vi "Build Wiring Spec.vi"(8 "error in (no error)":errorcluster, 10 "References":T1) -> (0 "error out":errorcluster, 4 "Wiring Spec":T2)   [LabVIEW 2023, in "Message Maker.lvclass"]
doc: "Figures out the wiring spec for the new message. This wiring spec is used to build the new message\n\nAuthor: Derek Trepanier\nCopyright: MGI 2015"
uses:
  Message Maker.lvclass
  Message Maker.lvclass/Message Maker.ctl
  <vilib>/Utility/VariantDataType/VariantType.lvlib
  Wiring Spec.ctl
  Connector Pane Position.ctl
  Scripting Refs.ctl
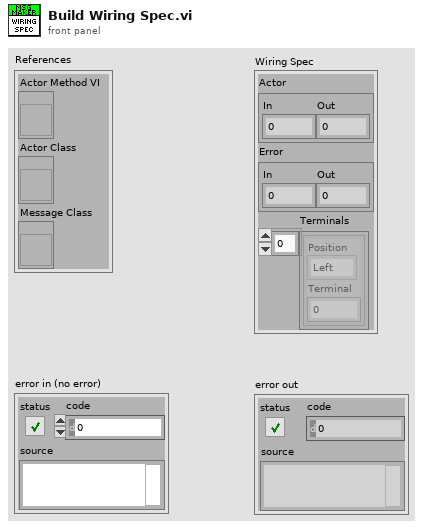
[diagram p1: front panel]
types:
  T1 = typedef "Message Maker.lvclass/Scripting Refs.ctl" = cluster{"Actor Method VI":refnum<vi>, "Actor Class":refnum<vi>, "Message Class":refnum<vi>}
  T2 = typedef "Message Maker.lvclass/Wiring Spec.ctl" = cluster{"Actor":cluster{"In":i32, "Out":i32}, "Error":cluster{"In":i32, "Out":i32}, "Terminals":cluster{"Position":T3, "Terminal":i32}[]}
  T3 = typedef "Message Maker.lvclass/Connector Pane Position.ctl" = enum16{"Left", "Top", "Bottom", "Right"}
  T4 = cluster{"Actor":cluster{"In":i32, "Out":i32}, "Error":cluster{"In":i32, "Out":i32}, "Left":cluster{"Position":i16, "Terminal":i32}[], "Bottom":cluster{"Position":i16, "Terminal":i32}[], "Right":cluster{"Position":i16, "Terminal":i32}[], "Top":cluster{"Position":i16, "Terminal":i32}[]}
  T5 = enum16{"Invalid Wire Rule", "Required", "Recommended", "Optional", "Dynamic Dispatch"}[]
  T6 = typedef "LVRectTypeDef.ctl" = cluster{"Left":i16, "Top":i16, "Right":i16, "Bottom":i16}
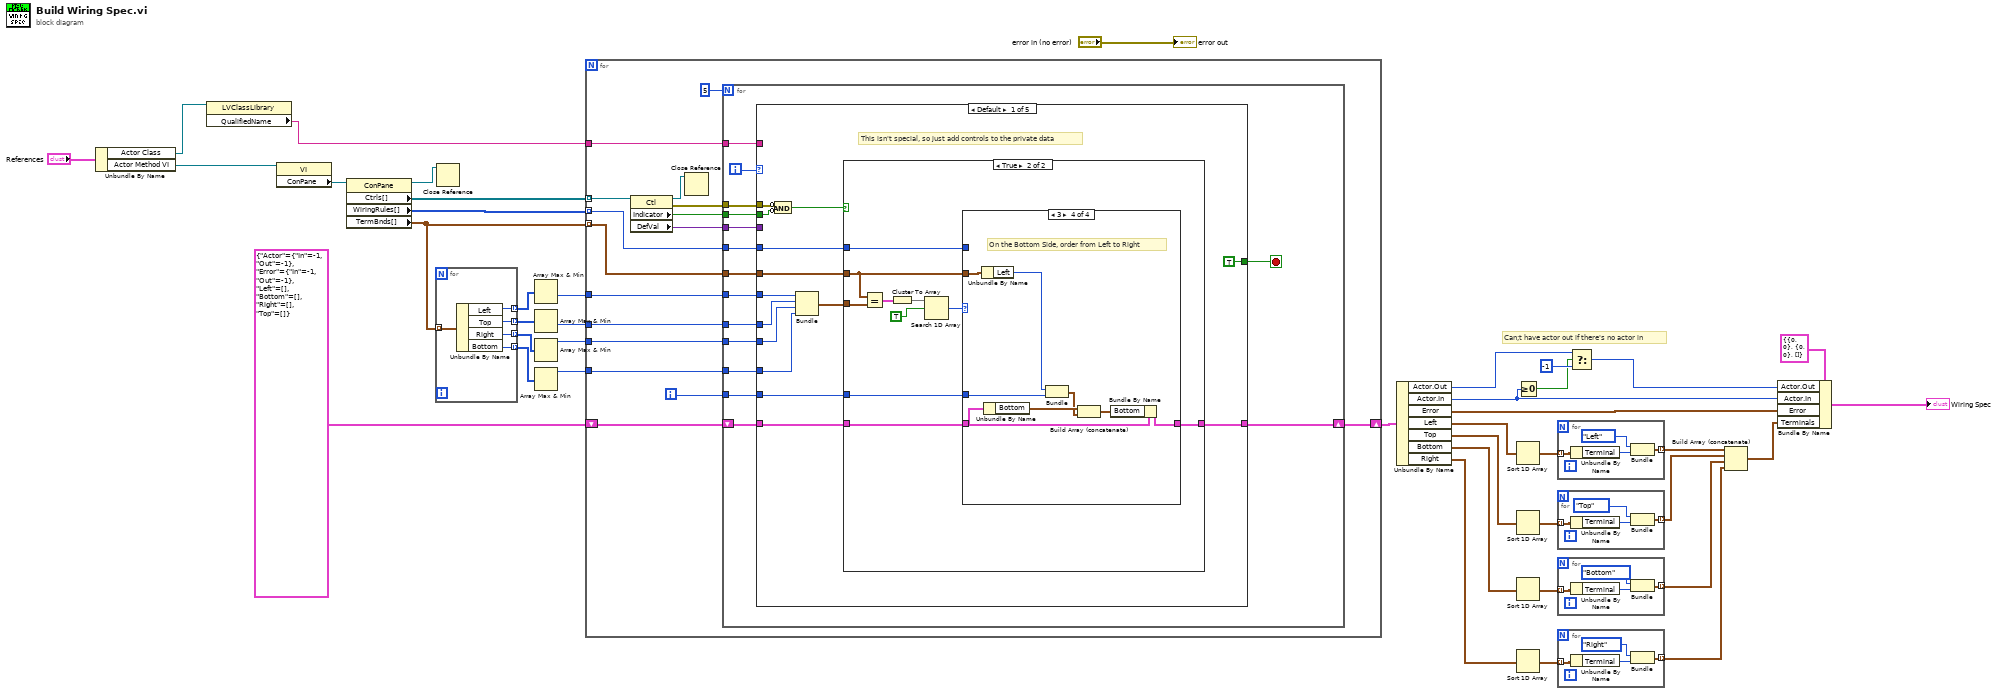
[diagram p0: block diagram]
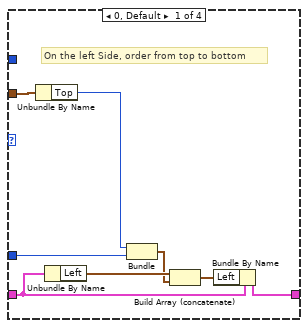
[diagram p3: hidden frame]
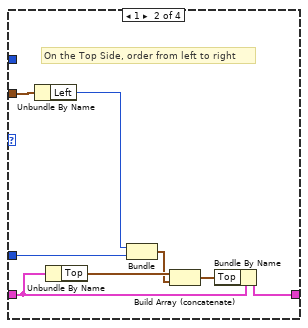
[diagram p4: hidden frame]
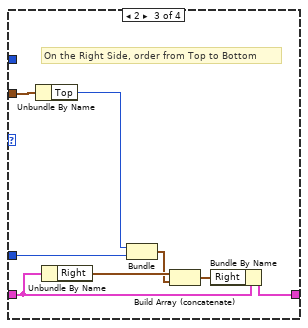
[diagram p5: hidden frame]
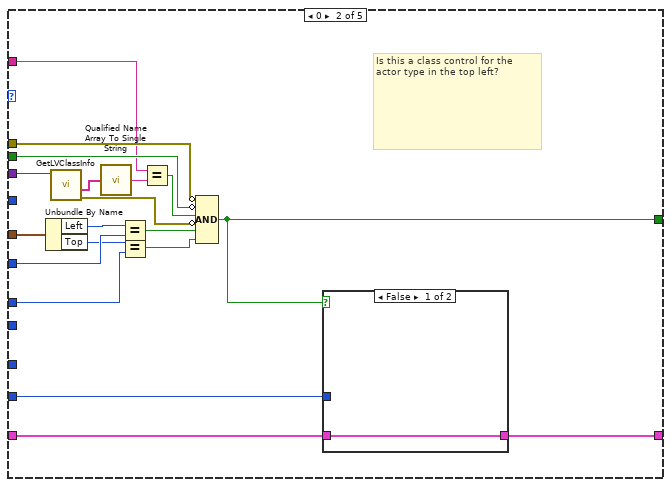
[diagram p6: hidden frame]
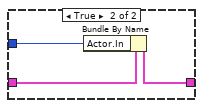
[diagram p7: hidden frame]
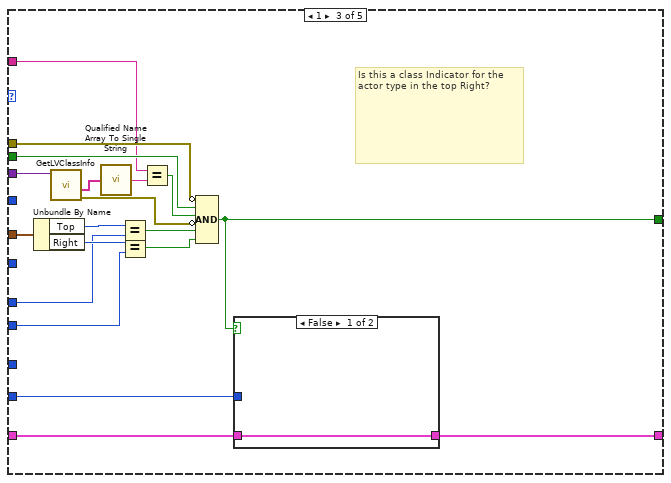
[diagram p8: hidden frame]
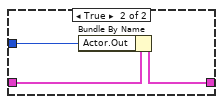
[diagram p9: hidden frame]
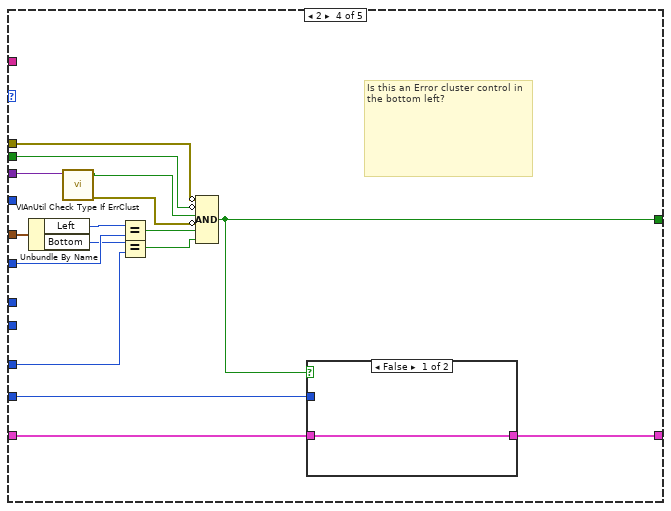
[diagram p10: hidden frame]
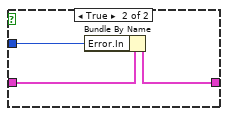
[diagram p11: hidden frame]
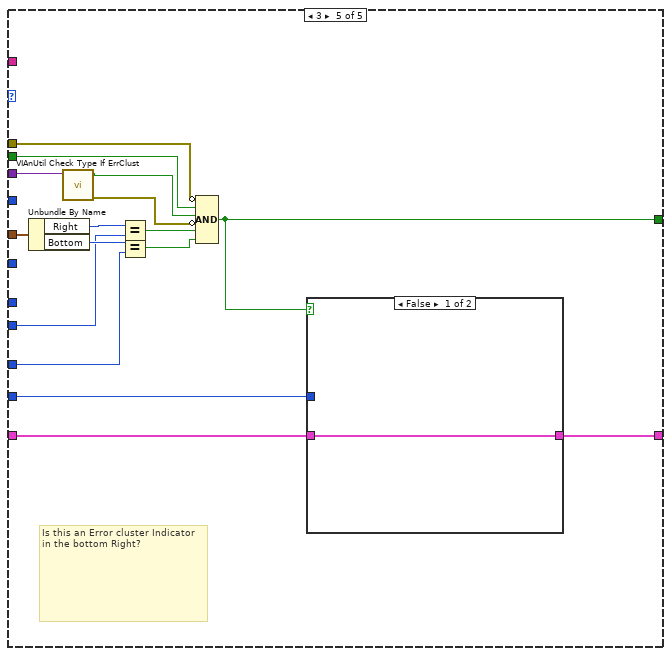
[diagram p12: hidden frame]
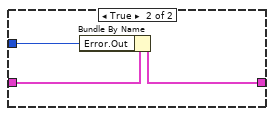
[diagram p13: hidden frame]
diagram:
  # "Can;t have actor out if there's no actor in"
  n1 = Unbundle By Name("References") -> ("Actor Class"=w4:refnum<vi>, "Actor Method VI"=w2:refnum<vi>)
  n2 = property class="LVClassLibrary"(reference=w4) -> ("QualifiedName"=w3:string)  [unwired: 1 in, 2 out]
  n3 = property class="VI"(reference=w2) -> ("ConPane"=w41:refnum<vi>)  [unwired: 1 in, 2 out]
  n4 = property class="ConPane"(reference=w41) -> (reference out=w30:refnum<vi>, "Ctrls[]"=w40:refnum<vi>[], "WiringRules[]"=w17:T5, "TermBnds[]"=w39:T6[])  [unwired: 1 in, 1 out]
  n5 = for {
    tunnel: w39 -> [w46] mode=indexing
    tunnel: [w45] -> w38 mode=indexing
    tunnel: [w44] -> w37 mode=indexing
    tunnel: [w43] -> w36 mode=indexing
    tunnel: [w42] -> w35 mode=indexing
    n6 = Unbundle By Name(w46) -> ("Left"=w45:i16, "Top"=w44:i16, "Right"=w43:i16, "Bottom"=w42:i16)
  }
  n7 = Close Reference(reference=w30) -> ()  [unwired: 1 in, 1 out]
  n8 = Array Max & Min(array=w38) -> (min value=w34:i16)  [unwired: 3 out]
  n9 = Array Max & Min(array=w37) -> (min value=w33:i16)  [unwired: 3 out]
  n10 = Array Max & Min(array=w36) -> (max value=w32:i16)  [unwired: 3 out]
  n11 = Array Max & Min(array=w35) -> (max value=w31:i16)  [unwired: 3 out]
  n12 = for {
    tunnel: w40 -> [w62] mode=indexing
    tunnel: w39 -> [w60] mode=indexing
    tunnel: w34 -> [w59]
    tunnel: w33 -> [w58]
    tunnel: w32 -> [w51]
    tunnel: w31 -> [w52]
    tunnel: w3 -> [w54]
    shift-right: [w48] -> w28
    shift-left: T4 {"Actor"={"In"=-1, "Out"=-1}, "Error"={"In"=-1, "Out"=-1}, "Left"=[], "Bottom"=[], "Right"=[], "Top"=[]} -> [w49]
    tunnel: w17 -> [w47] mode=indexing
    i -> [w53]
    # "Find Top Left, Bottom left controls AND\nTop Right and bottom right Indicators"
    n13 = property class="Ctl"(reference=w62) -> (reference out=w50:refnum<vi>, error out=w57:errorcluster, "Indicator"=w56:bool, "DefVal"=w55:variant)  [unwired: 1 in]
    n14 = Close Reference(reference=w50) -> ()  [unwired: 1 in, 1 out]
    n15 = for {
      N: 5 -> [_]
      tunnel: w60 -> [w76]
      shift-right: [w67] -> w48
      shift-left: w49 -> [w75]
      tunnel: w59 -> [w74]
      tunnel: w58 -> [w73]
      tunnel: w57 -> [w72]
      tunnel: w56 -> [w71]
      tunnel: w55 -> [w70]
      tunnel: w54 -> [w69]
      tunnel: w53 -> [w68]
      tunnel: w52 -> [w66]
      tunnel: w51 -> [w65]
      tunnel: w47 -> [w63]
      i -> [w77]
      stop <- w64 stop-if-true
      n16 = case shown="Default" w77 {
        tunnel: w76 -> [w84 w153 w176 w196 w216]
        tunnel: w75 -> [w91 w138 w163 w182 w202]
        tunnel: w74 -> [w83 w151 _ w194 _]
        tunnel: w73 -> [w82 w149 w161 _ _]
        tunnel: w72 -> [w89 w148 w173 w192 w213]
        tunnel: w71 -> [w88 w147 w172 w191 w212]
        tunnel: w70 -> [_ w143 w168 w187 w208]
        tunnel: w69 -> [_ w140 w165 _ _]
        tunnel: w68 -> [w86 w137 w162 w188 w209]
        tunnel: [w90 w135 w158 w181 w201] -> w67
        tunnel: w66 -> [w80 _ _ w184 w205]
        tunnel: w65 -> [w81 _ w160 _ w204]
        tunnel: [TRUE w136 w159 w183 w203] -> w64
        tunnel: w63 -> [w78 _ _ _ _]
        frame Default {
          # "This isn't special, so just add controls to the private data"
          n17 = Compound Arithmetic op=AND(invert w89, invert w88) -> (w87:bool)
          n18 = Bundle(w83, w82, w81, w80) -> (w79:cluster{i16, i16, i16, i16})  [unwired: 1 in]
          n19 = case shown="True" w87 {
            tunnel: w91 -> [w92 w96]
            tunnel: [w92 w94] -> w90
            tunnel: w86 -> [_ w95]
            tunnel: w84 -> [_ w97]
            tunnel: w79 -> [_ w102]
            tunnel: w78 -> [_ w93]
            frame False {
            }
            frame True {
              n20 = Equal?(x=w97, y=w102) -> (x = y?=w101:cluster{bool, bool, bool, bool})
              n21 = Cluster To Array(cluster=w101) -> (array=w100:bool[])
              n22 = Search 1D Array(1D array=w100, element=TRUE) -> (index of element=w98:i32)  [unwired: 1 in]
              n23 = case shown="3" w98 {
                tunnel: w97 -> [w110 w118 w126 w134]
                tunnel: w96 -> [w107 w115 w123 w131]
                tunnel: w95 -> [w108 w116 w124 w132]
                tunnel: [w104 w112 w120 w128] -> w94
                tunnel: w93 -> [_ _ _ _]
                frame 0, Default {
                  # "On the left Side, order from top to bottom"
                  n24 = Unbundle By Name(w110) -> ("Top"=w109:i16)
                  n25 = Unbundle By Name(w107) -> ("Left"=w106:cluster{"Position":i16, "Terminal":i32}[])
                  n26 = Bundle("Top"=w109, w108) -> (w105:cluster{"Top":i16, i32})  [unwired: 1 in]
                  n27 = Build Array (concatenate)(w106, w105) -> (w103:cluster{"Top":i16, "Terminal":i32}[])
                  n28 = Bundle By Name(cluster=w107, "Left"=w103) -> (w104:T4)
                }
                frame 1 {
                  # "On the Top Side, order from left to right"
                  n29 = Unbundle By Name(w118) -> ("Left"=w117:i16)
                  n30 = Unbundle By Name(w115) -> ("Top"=w114:cluster{"Position":i16, "Terminal":i32}[])
                  n31 = Bundle("Left"=w117, w116) -> (w113:cluster{"Left":i16, i32})  [unwired: 1 in]
                  n32 = Build Array (concatenate)(w114, w113) -> (w111:cluster{"Left":i16, "Terminal":i32}[])
                  n33 = Bundle By Name(cluster=w115, "Top"=w111) -> (w112:T4)
                }
                frame 2 {
                  # "On the Right Side, order from Top to Bottom"
                  n34 = Unbundle By Name(w126) -> ("Top"=w125:i16)
                  n35 = Unbundle By Name(w123) -> ("Right"=w122:cluster{"Position":i16, "Terminal":i32}[])
                  n36 = Bundle("Top"=w125, w124) -> (w121:cluster{"Top":i16, i32})  [unwired: 1 in]
                  n37 = Build Array (concatenate)(w122, w121) -> (w119:cluster{"Top":i16, "Terminal":i32}[])
                  n38 = Bundle By Name(cluster=w123, "Right"=w119) -> (w120:T4)
                }
                frame 3 {
                  # "On the Bottom Side, order from Left to Right"
                  n39 = Unbundle By Name(w134) -> ("Left"=w133:i16)
                  n40 = Unbundle By Name(w131) -> ("Bottom"=w130:cluster{"Position":i16, "Terminal":i32}[])
                  n41 = Bundle("Left"=w133, w132) -> (w129:cluster{"Left":i16, i32})  [unwired: 1 in]
                  n42 = Build Array (concatenate)(w130, w129) -> (w127:cluster{"Left":i16, "Terminal":i32}[])
                  n43 = Bundle By Name(cluster=w131, "Bottom"=w127) -> (w128:T4)
                }
              }
            }
          }
        }
        frame 0 {
          # "Is this a class control for the actor type in the top left?"
          # "Top Left Actor Class Ctrl?"
          n44 = Unbundle By Name(w153) -> ("Left"=w152:i16, "Top"=w150:i16)
          n45 = call <vilib>:"GetLVClassInfo.vi"("Variant"=w143) -> ("error out"=w142:errorcluster, "Fully Qualified LV Class Name"=w144:string[])  [unwired: 8 in, 1 out]
          n46 = call <vilib>:"Qualified Name Array To Single String.vi"("Fully Qualified Array"=w144) -> ("Fully Qualified String"=w141:string)
          n47 = Equal?(x=w152, y=w151) -> (x = y?=w146:bool)
          n48 = Equal?(x=w150, y=w149) -> (x = y?=w145:bool)
          n49 = Equal?(x=w140, y=w141) -> (x = y?=w139:bool)
          n50 = Compound Arithmetic op=AND(invert w148, invert w147, w139, invert w142, w146, w145) -> (w136:bool)
          n51 = case shown="False" w136 {
            tunnel: w138 -> [w154 w155]
            tunnel: w137 -> [_ w156]
            tunnel: [w154 w157] -> w135
            frame False {
            }
            frame True {
              n52 = Bundle By Name(cluster=w155, "Actor.In"=w156) -> (w157:T4)
            }
          }
        }
        frame 1 {
          # "Is this a class Indicator for the actor type in the top Right?"
          # "Top Left Actor Class Ctrl?"
          n53 = Unbundle By Name(w176) -> ("Top"=w175:i16, "Right"=w174:i16)
          n54 = call <vilib>:"GetLVClassInfo.vi"("Variant"=w168) -> ("error out"=w167:errorcluster, "Fully Qualified LV Class Name"=w169:string[])  [unwired: 8 in, 1 out]
          n55 = call <vilib>:"Qualified Name Array To Single String.vi"("Fully Qualified Array"=w169) -> ("Fully Qualified String"=w166:string)
          n56 = Equal?(x=w175, y=w161) -> (x = y?=w171:bool)
          n57 = Equal?(x=w174, y=w160) -> (x = y?=w170:bool)
          n58 = Equal?(x=w165, y=w166) -> (x = y?=w164:bool)
          n59 = Compound Arithmetic op=AND(invert w173, w172, w164, invert w167, w171, w170) -> (w159:bool)
          n60 = case shown="False" w159 {
            tunnel: w163 -> [w177 w178]
            tunnel: w162 -> [_ w179]
            tunnel: [w177 w180] -> w158
            frame False {
            }
            frame True {
              n61 = Bundle By Name(cluster=w178, "Actor.Out"=w179) -> (w180:T4)
            }
          }
        }
        frame 2 {
          # "Is this an Error cluster control in the bottom left?"
          # "Top Left Actor Class Ctrl?"
          n62 = Unbundle By Name(w196) -> ("Left"=w195:i16, "Bottom"=w193:i16)
          n63 = call <vilib>:"VIAnUtil Check Type If ErrClust.vi"("Data In"=w187) -> ("error out"=w186:errorcluster, "IsErrClust?"=w185:bool)  [unwired: 9 in]
          n64 = Equal?(x=w195, y=w194) -> (x = y?=w190:bool)
          n65 = Equal?(x=w193, y=w184) -> (x = y?=w189:bool)
          n66 = Compound Arithmetic op=AND(invert w192, invert w191, w185, invert w186, w190, w189) -> (w183:bool)
          n67 = case shown="False" w183 {
            tunnel: w188 -> [_ w199]
            tunnel: [w197 w200] -> w181
            tunnel: w182 -> [w197 w198]
            frame False {
            }
            frame True {
              n68 = Bundle By Name(cluster=w198, "Error.In"=w199) -> (w200:T4)
            }
          }
        }
        frame 3 {
          # "Is this an Error cluster Indicator in the bottom Right?"
          # "Top Left Actor Class Ctrl?"
          n69 = Unbundle By Name(w216) -> ("Right"=w215:i16, "Bottom"=w214:i16)
          n70 = call <vilib>:"VIAnUtil Check Type If ErrClust.vi"("Data In"=w208) -> ("error out"=w207:errorcluster, "IsErrClust?"=w206:bool)  [unwired: 9 in]
          n71 = Equal?(x=w215, y=w204) -> (x = y?=w211:bool)
          n72 = Equal?(x=w214, y=w205) -> (x = y?=w210:bool)
          n73 = Compound Arithmetic op=AND(invert w213, w212, w206, invert w207, w211, w210) -> (w203:bool)
          n74 = case shown="False" w203 {
            tunnel: w209 -> [_ w219]
            tunnel: [w217 w220] -> w201
            tunnel: w202 -> [w217 w218]
            frame False {
            }
            frame True {
              n75 = Bundle By Name(cluster=w218, "Error.Out"=w219) -> (w220:T4)
            }
          }
        }
      }
    }
  }
  n76 = Unbundle By Name(w28) -> ("Actor.Out"=w24:i32, "Actor.In"=w21:i32, "Error"=w26:cluster{"In":i32, "Out":i32}, "Left"=w20:cluster{"Position":i16, "Terminal":i32}[], "Top"=w13:cluster{"Position":i16, "Terminal":i32}[], "Bottom"=w12:cluster{"Position":i16, "Terminal":i32}[], "Right"=w11:cluster{"Position":i16, "Terminal":i32}[])
  n77 = Sort 1D Array(array=w20) -> (sorted array=w19:cluster{"Position":i16, "Terminal":i32}[])
  n78 = Sort 1D Array(array=w13) -> (sorted array=w16:cluster{"Position":i16, "Terminal":i32}[])
  n79 = Sort 1D Array(array=w12) -> (sorted array=w15:cluster{"Position":i16, "Terminal":i32}[])
  n80 = Sort 1D Array(array=w11) -> (sorted array=w14:cluster{"Position":i16, "Terminal":i32}[])
  n81 = Greater Or Equal To 0?(x=w21) -> (x >= 0?=w22:bool)
  n82 = for {
    tunnel: w19 -> [w224] mode=indexing
    tunnel: [w221] -> w10 mode=indexing
    n83 = Unbundle By Name(w224) -> ("Terminal"=w222:i32)
    n84 = Bundle("Position"=Connector_Pane_Position."Left", "Terminal"=w222) -> (w221:cluster{"Position":T3, "Terminal":i32})  [unwired: 1 in]
  }
  n85 = for {
    tunnel: w16 -> [w228] mode=indexing
    tunnel: [w225] -> w9 mode=indexing
    n86 = Unbundle By Name(w228) -> ("Terminal"=w226:i32)
    n87 = Bundle("Position"=Connector_Pane_Position."Top", "Terminal"=w226) -> (w225:cluster{"Position":T3, "Terminal":i32})  [unwired: 1 in]
  }
  n88 = for {
    tunnel: w15 -> [w232] mode=indexing
    tunnel: [w229] -> w8 mode=indexing
    n89 = Unbundle By Name(w232) -> ("Terminal"=w230:i32)
    n90 = Bundle("Position"=Connector_Pane_Position."Bottom", "Terminal"=w230) -> (w229:cluster{"Position":T3, "Terminal":i32})  [unwired: 1 in]
  }
  n91 = for {
    tunnel: w14 -> [w236] mode=indexing
    tunnel: [w233] -> w7 mode=indexing
    n92 = Unbundle By Name(w236) -> ("Terminal"=w234:i32)
    n93 = Bundle("Position"=Connector_Pane_Position."Right", "Terminal"=w234) -> (w233:cluster{"Position":T3, "Terminal":i32})  [unwired: 1 in]
  }
  n94 = Select(t=w24, s=w22, f=-1) -> (s? t:f=w25:i32)
  n95 = Build Array (concatenate)(w10, w9, w8, w7) -> (w6:cluster{"Position":T3, "Terminal":i32}[])
  n96 = Bundle By Name(cluster=T2 {"Actor"={"In"=0, "Out"=0}, "Error"={"In"=0, "Out"=0}, "Terminals"=[]} ("Wiring Spec"), "Actor.Out"=w25, "Actor.In"=w21, "Error"=w26, "Terminals"=w6) -> (→"Wiring Spec":T2)
  "error out" <- "error in (no error)"
